vi "Compute DistanceTo AprilTag.vi"(6 "Robot Calibration Cluster":T1={"Camera Height on robot (in)"=34.5, "Camera Angle on the robot (deg)"=28.3, "Camera FOV Top to Bottom View Angle (deg)"=0.946, "Camera FOV Left to Right View Angle (deg)"=26.5, "Target size (in)"=6.5, "Focal Length (mm)"=10.0} {"Camera FOV Left to Right View Angle (deg)" format="%#_13g"; "Focal Length (mm)" format="%#_13g"; "Target size (in)" format="%#_13g"; "Camera FOV Top to Bottom View Angle (deg)" format="%#_13g"; "Camera Angle on the robot (deg)" format="%#_13g"; "Camera Height on robot (in)" format="%#_13g"}, 8 "results":T2={"diameter points"={"first point"={"x"=0.0, "y"=0.0}, "projected point"={"x"=0.0, "y"=0.0}}, "normalized center"={"x"=0.0, "y"=0.0}, "Overall Score"=0.0, "Distance (ft)"=0.0, "Offset Angle"=0.0, "Tag corner points"=[], "Tag Center"={"X"=0.0, "Y"=0.0}, "Tag Yaw"=0.0, "Tag Pitch"=0.0, "Target Roll (deg)"=0.0, "AprilTag Number"=68, "homography matrix"=[]} {"Tag Center"."Y" format="%0.2f"; "Tag Center"."X" format="%0.2f"}, 11 "Image Src":T3) -> (0 "results out":T2={"diameter points"={"first point"={"x"=0.0, "y"=0.0}, "projected point"={"x"=0.0, "y"=0.0}}, "normalized center"={"x"=0.0, "y"=0.0}, "Overall Score"=0.0, "Distance (ft)"=0.0, "Offset Angle"=0.0, "Tag corner points"=[], "Tag Center"={"X"=0.0, "Y"=0.0}, "Tag Yaw"=0.0, "Tag Pitch"=0.0, "Target Roll (deg)"=0.0, "AprilTag Number"=68, "homography matrix"=[]} {"Tag Center"."Y" format="%0.2f"; "Tag Center"."X" format="%0.2f"}, 1 "Target Yaw (deg)":dbl, 2 "Offset Angle":dbl=569.258018632146, 3 "Image Dst Out":T3, 4 "Distance from target (in)":dbl=116.40675998176638 format="%.2f", 5 "Target Pitch (deg)":dbl)   [LabVIEW 2025]
doc: "Using the camera lens information and the real world size of the target, use trig and ratios to determine the distance to the target. Also returns the location relative to the image center in a (-1 , 1) coordinate system that may be useful for steering the robot."
uses:
  <vilib>/vision/Image Controls.llb/IMAQ Image.ctl
  AprilTag Target Fields.ctl
  Camera Info.ctl
panel:
  out "Target Roll (deg)":dbl
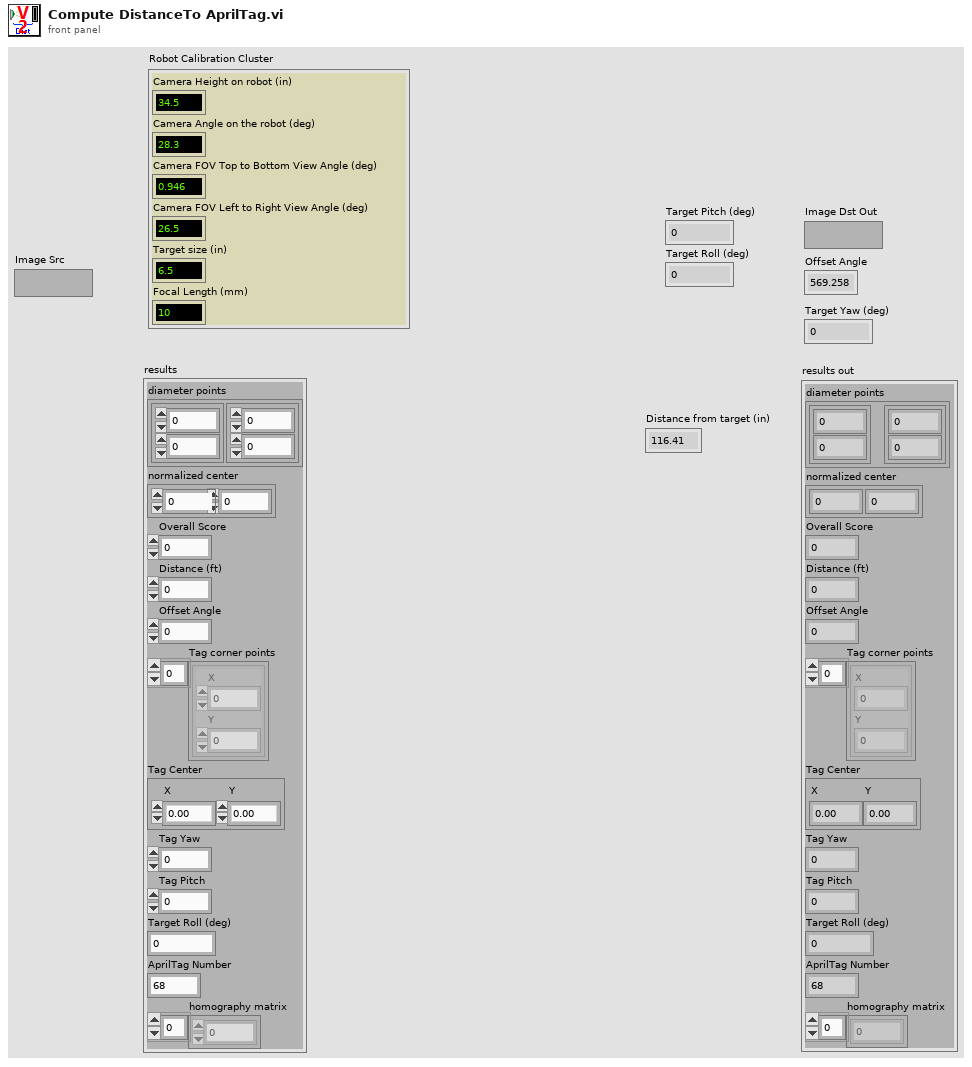
[diagram p1: front panel]
types:
  T1 = typedef "Camera Info.ctl" = cluster{"Camera Height on robot (in)":dbl, "Camera Angle on the robot (deg)":dbl, "Camera FOV Top to Bottom View Angle (deg)":dbl, "Camera FOV Left to Right View Angle (deg)":dbl, "Target size (in)":dbl, "Focal Length (mm)":dbl}
  T2 = typedef "AprilTag Target Fields.ctl" = cluster{"diameter points":cluster{"first point":cluster{"x":dbl, "y":dbl}, "projected point":cluster{"x":dbl, "y":dbl}}, "normalized center":cluster{"x":dbl, "y":dbl}, "Overall Score":dbl, "Distance (ft)":dbl, "Offset Angle":dbl, "Tag corner points":cluster{"X":dbl, "Y":dbl}[], "Tag Center":cluster{"X":dbl, "Y":dbl}, "Tag Yaw":dbl, "Tag Pitch":dbl, "Target Roll (deg)":dbl, "AprilTag Number":i32, "homography matrix":dbl[]}
  T3 = typedef "IMAQ Image.ctl" = refnum<image>
  T4 = cluster{"first point":cluster{"x":dbl, "y":dbl}, "projected point":cluster{"x":dbl, "y":dbl}}
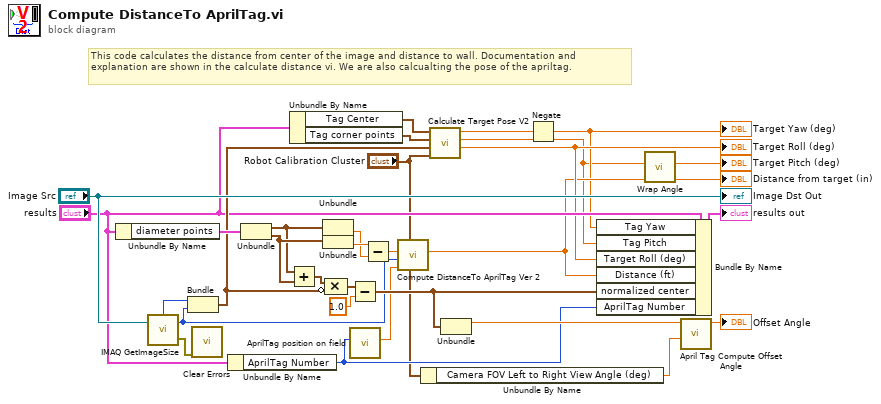
[diagram p0: block diagram]
diagram:
  # "This code calculates the distance from center of the image and distance to wall. Documentation and explanation are shown in the calculate distance vi. We are also calcualting the pose of the apriltag."
  n1 = Unbundle By Name("results") -> ("diameter points"=w14:T4)
  n2 = call "IMAQ GetImageSize"("Image"="Image Src") -> ("Y Resolution"=w21:i32, "X Resolution"=w22:i32, "error out"=w31:errorcluster)  [unwired: 3 in]
  n3 = Bundle("X Resolution"=w22, "Y Resolution"=w21) -> (w13:cluster{"X Resolution":i32, "Y Resolution":i32})  [unwired: 1 in]
  n4 = call <vilib>:"Clear Errors.vi"("error in (no error)"=w31) -> ()  [unwired: 5 in, 2 out]
  n5 = Unbundle By Name("results") -> ("AprilTag Number"=w9:i32)
  n6 = Unbundle(w14) -> ("first point"=w15:cluster{"x":dbl, "y":dbl}, "projected point"=w20:cluster{"x":dbl, "y":dbl})
  n7 = Add(x=w15, y=w20) -> (x+y=w27:cluster{"x":dbl, "y":dbl})
  n8 = Unbundle By Name("results") -> ("Tag Center"=w11:cluster{"X":dbl, "Y":dbl}, "Tag corner points"=w12:cluster{"X":dbl, "Y":dbl}[])
  n9 = Unbundle(w15) -> ("y"=w17:dbl)  [unwired: 1 out]
  n10 = Unbundle(w20) -> ("y"=w18:dbl)  [unwired: 1 out]
  n11 = Compound Arithmetic op=MULTIPLY(w27, invert w13) -> (w28:cluster{dbl, dbl})
  n12 = Subtract(x=w28, y=1.0) -> (x-y=w25:cluster{dbl, dbl})
  n13 = call "AprilTag position on field.vi"("AprilTag Number"=w9) -> ("Target height to center (in)"=w19:dbl)  [unwired: 10 in]
  n14 = Subtract(x=w18, y=w17) -> (x-y=w16:dbl)
  n15 = call "Compute DistanceTo AprilTag Ver 2.vi"("Robot Calibration Cluster"="Robot Calibration Cluster", "Height to center of target from floor (hp (in))"=w19, "Screen resolution pixels Height (Ry)"=w21, "Target Vertical pixels bottom - top (pixels)"=w16) -> ("Distance from target to camera (in)"=w4:dbl)  [unwired: 7 in]
  "Distance from target (in)" <- w4
  n16 = Unbundle By Name("Robot Calibration Cluster") -> ("Camera FOV Left to Right View Angle (deg)"=w7:dbl)
  n17 = call "Calculate Target Pose V2.vi"("Robot Calibration Cluster"="Robot Calibration Cluster", "Camera Resolution"=w13, "Corners"=w12, "Target Center"=w11) -> ("Roll"=w8:dbl, "Pitch"=w2:dbl, "Yaw"=w6:dbl)  [unwired: 4 in, 1 out]
  "Target Roll (deg)" <- w8
  n18 = Unbundle(w25) -> (w24:dbl)  [unwired: 1 out]
  n19 = Negate(x=w6) -> (-x=w3:dbl)
  "Target Yaw (deg)" <- w3
  n20 = Bundle By Name(cluster="results", "Tag Yaw"=w3, "Tag Pitch"=w2, "Target Roll (deg)"=w8, "Distance (ft)"=w4, "normalized center"=w25, "AprilTag Number"=w9) -> (→"results out":T2)
  n21 = call "Wrap Angle.vi"("Target Pitch (deg)"=w2) -> ("Correct Pitch"=→"Target Pitch (deg)":dbl)  [unwired: 10 in]
  n22 = call "April Tag Compute Offset Angle.vi"("Field of view"=w7, "Offset Normilized"=w24) -> ("Offset Angle"=→"Offset Angle":dbl)  [unwired: 9 in]
  "Image Dst Out" <- "Image Src"
